vi "Lookup Service Port.vi"(8 "error in (no error)":errorcluster, 9 "Service Type":T3, 10 "node_id":u32, 11 "NodeDiscovery in":refnum<class "DiscoveryService.lvclass">) -> (0 "error out":errorcluster, 1 "port":i32, 2 "Node":T1, 3 "NodeDiscovery out":refnum<class "DiscoveryService.lvclass">)   [LabVIEW 2020, in "Vecto.lvlib" / "DiscoveryService.lvclass"]
uses:
  DiscoveryService.lvclass
  lv-volatus/messages/ServiceType/Enumeration.ctl
  lv-volatus/messages/Discovery/Data.ctl
  lv-volatus/messages/Service/Data.ctl
  lv-volatus/messages/ServiceType/ServiceType.lvlib
  lv-volatus/messages/Service/Service.lvlib
  lv-volatus/messages/Discovery/Discovery.lvlib
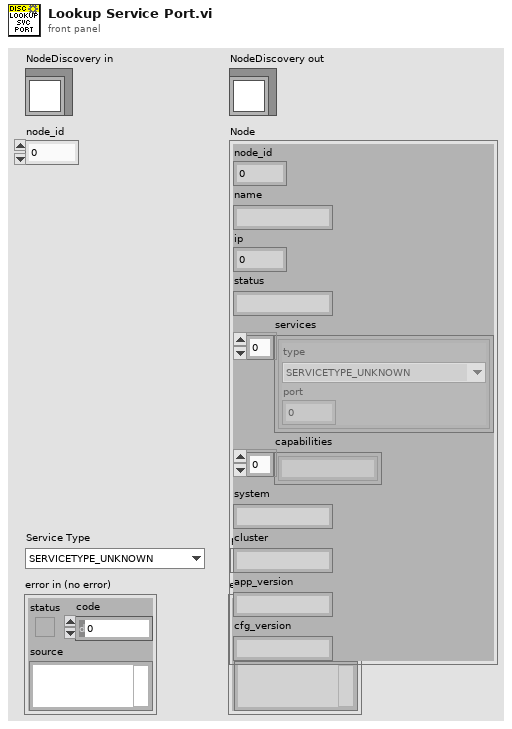
[diagram p1: front panel]
types:
  T1 = typedef "Discovery.lvlib/Data.ctl" = cluster{"node_id":u32, "name":string, "ip":u32, "status":string, "services":T2[], "capabilities":string[], "system":string, "cluster":string, "app_version":string, "cfg_version":string}
  T2 = typedef "Service.lvlib/Data.ctl" = cluster{"type":T3, "port":i32}
  T3 = typedef "ServiceType.lvlib/Enumeration.ctl" = enum16{"SERVICETYPE_UNKNOWN", "SERVICETYPE_TCPSERVER", "SERVICETYPE_HTTPSERVER"}
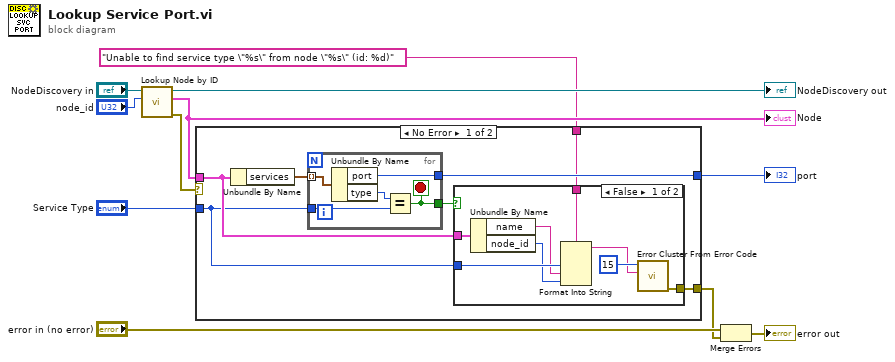
[diagram p0: block diagram]
diagram:
  n1 = call "Lookup Node by ID.vi"("node_id"="node_id", "DiscoveryService in"="NodeDiscovery in") -> ("error out"=w7:errorcluster, "Node"=w6:T1, "DiscoveryService out"=→"NodeDiscovery out":refnum<class "DiscoveryService.lvclass">)  [unwired: 7 in]
  "Node" <- w6
  n2 = case shown="No Error" w7 {
    selector: w7 -> [_ w32]
    tunnel: w6 -> [w15 _]
    tunnel: "Service Type" -> [w13 _]
    tunnel: [w17 _] -> w4
    tunnel: "Unable to find service type \"%s\" from node \"%s\" (id: %d)" -> [w14 _]
    tunnel: [w12 w32] -> w1
    frame No Error {
      n3 = Unbundle By Name(w15) -> ("services"=w18:T2[])
      n4 = for {
        tunnel: w18 -> [w31] mode=indexing
        tunnel: w13 -> [w29]
        tunnel: [w28] -> w17
        tunnel: [w27] -> w16
        stop <- w27 stop-if-true
        n5 = Unbundle By Name(w31) -> ("port"=w28:i32, "type"=w30:T3)
        n6 = Equal?(x=w30, y=w29) -> (x = y?=w27:bool)
      }
      n7 = case shown="False" w16 {
        tunnel: w15 -> [w25 _]
        tunnel: w14 -> [w24 _]
        tunnel: w13 -> [w23 _]
        tunnel: [w19 _] -> w12
        frame False {
          n8 = Unbundle By Name(w25) -> ("name"=w21:string, "node_id"=w22:u32)
          n9 = Format Into String(format string=w24, w23, w21, w22) -> (resulting string=w20:string)  [unwired: 2 in, 1 out]
          n10 = call <vilib>:"Error Cluster From Error Code.vi"("error message (\"\")"=w20, "error code (0)"=15) -> ("error out"=w19:errorcluster)  [unwired: 7 in]
        }
        frame True {
        }
      }
    }
    frame Error {
    }
  }
  "port" <- w4
  n11 = Merge Errors("error in (no error)", w1) -> (→"error out":errorcluster)
